vi "System und Gaseinstellung V2 - Kopie.vi"() -> ()   [LabVIEW 2020, in "System Einstellungen V2.lvlib"]
uses:
  System Einstellungen V2.lvlib
  Visualisierungs Elemente/String - Eingabefeld.ctl
  Gasflasche.ctl
  Gasflaschenkomponente.ctl
  Traegergas.ctl
  Aktion FGV Gasbottledefinition.ctl
  Allgemein/allgemeine Sub-VIs.lvlib
panel:
  in  "Update Gas Selects":bool caption="Schaltfläche"
  in  "Registerkartenelement":T1(tab)
  in  "Gasflaschen Liste Pfad":path caption="Gasbottle List File Path"
  in  "Gasflaschen Maske leeren":bool caption="Schaltfläche"
  in  "Gasflasche löschen":bool caption="Schaltfläche"
  in  "Gasflsche einfügen":bool caption="Schaltfläche"
  in  "Gasflasche ändern":bool caption="Schaltfläche"
  in  "Trägergas":T2="N2" caption="Carrier Gas"
  in  "Komponente 5":T3={"Gasauswahl"="", "Konzentration SOLL"=0.0, "Konzentration IST"=0.0, "Einheit"="ppm", "Genauigkeit"=0.0} caption="Component 5" {"Konzentration SOLL" format="%#.4f"; "Konzentration IST" format="%#.4f"; "Genauigkeit" format="%#.1f"}
  in  "Komponente 4":T3={"Gasauswahl"="", "Konzentration SOLL"=0.0, "Konzentration IST"=0.0, "Einheit"="ppm", "Genauigkeit"=0.0} caption="Component 4" {"Konzentration SOLL" format="%#.4f"; "Konzentration IST" format="%#.4f"; "Genauigkeit" format="%#.1f"}
  in  "Komponente 3":T3={"Gasauswahl"="", "Konzentration SOLL"=0.0, "Konzentration IST"=0.0, "Einheit"="ppm", "Genauigkeit"=0.0} caption="Component 3" {"Konzentration SOLL" format="%#.4f"; "Konzentration IST" format="%#.4f"; "Genauigkeit" format="%#.1f"}
  in  "Komponente 2":T3={"Gasauswahl"="", "Konzentration SOLL"=0.0, "Konzentration IST"=0.0, "Einheit"="ppm", "Genauigkeit"=0.0} caption="Component 2" {"Konzentration SOLL" format="%#.4f"; "Konzentration IST" format="%#.4f"; "Genauigkeit" format="%#.1f"}
  in  "Komponente 1":T3={"Gasauswahl"="", "Konzentration SOLL"=0.0, "Konzentration IST"=0.0, "Einheit"="ppm", "Genauigkeit"=0.0} caption="Component 1" {"Konzentration SOLL" format="%#.4f"; "Konzentration IST" format="%#.4f"; "Genauigkeit" format="%#.1f"}
  in  "Gasflasche":T4={"Gasname für die Auswahl"="CH4", "Gasflaschennummer  (Zylinder)"="D15442589", "Chargennummer"="D15442589", "Volumen"="D15442589", "Herstelldatum"=timestamp(0 s since 1904-01-01), "Ablaufdatum"=timestamp(0 s since 1904-01-01)} {"Ablaufdatum" format="%<%d.%m.%Y>T"; "Herstelldatum" format="%<%d.%m.%Y>T"}
  in  "GF import":bool caption="Schaltfläche 2"
  in  "GF export":bool caption="Schaltfläche"
  in  "Gasflaschen Liste":i32(listbox) caption="List of Gasbottles"
  in  "Gas Eingabe":T5
  in  "Gas einfügen":bool caption="Schaltfläche"
  in  "Markiertes Gas löschen":bool caption="Schaltfläche"
  in  "Gasauswahl":i32(listbox) caption="Gasauswahl erstellte Gasflaschen"
  # "System Settings"
  # "Ziel: bei jeder PDF und Einstellung die Seriennummer automatisch laden oder auszuwählen zu können"
  # "Analysator Seriennummer Eintrag"
  # "Alte Systemeinstellungen (PopUp) übernehmen"
  # "Unsere derzeitige Calgas Einstellung fürs Kalibrieren\n\nEventuell Analyser Spalte wie LowNox"
  # "Gas"
  # "Nominal"
  # "Real"
  # "Unit"
  # "Accuracy %"
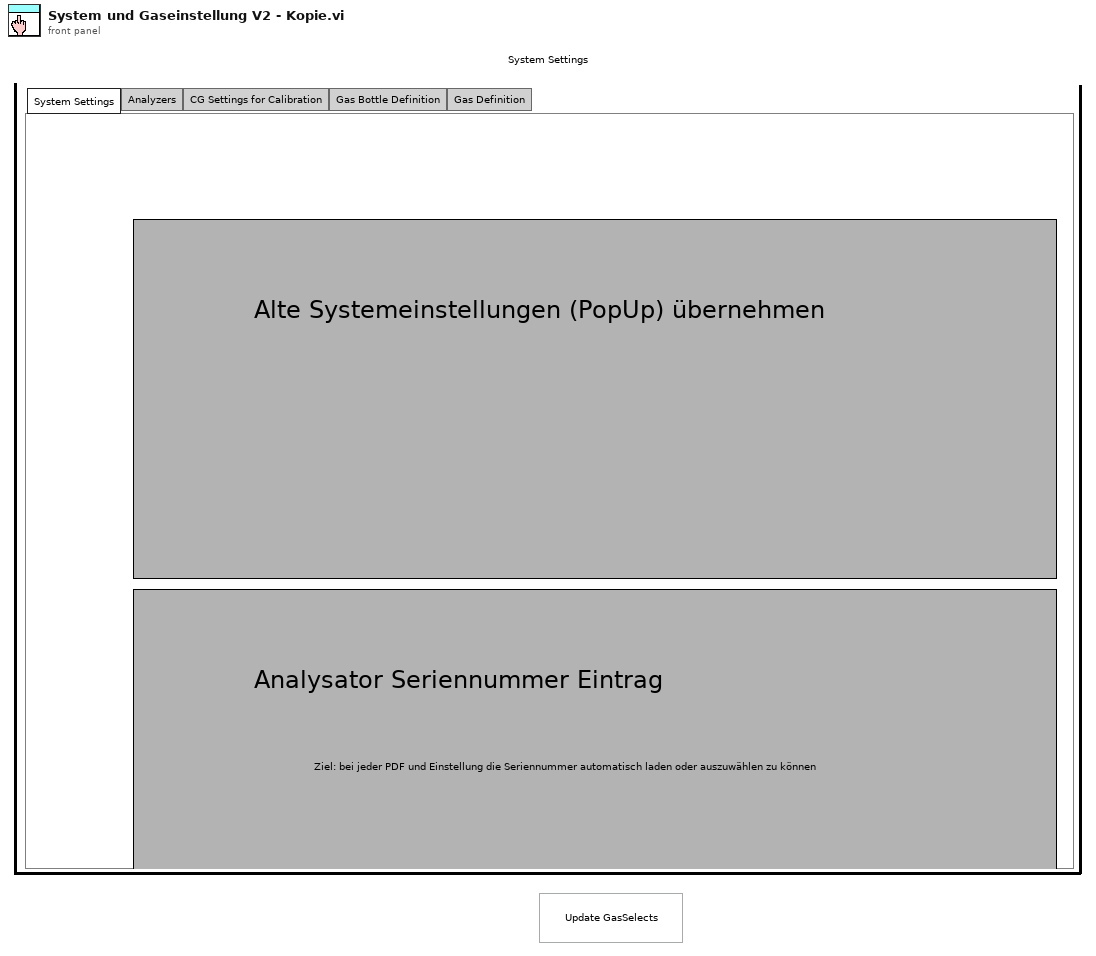
[diagram p1: front panel]
types:
  T1 = enum32{"Systemeinstellungen", "Analysatoren", "CG-Einstellung für Kalibrierung", "Gasflaschenkonfiguration", "Gasdefinition"}
  T2 = typedef "System Einstellungen V2.lvlib/Traegergas.ctl" = string
  T3 = typedef "System Einstellungen V2.lvlib/Gasflaschenkomponente.ctl" = cluster{"Gasauswahl":string, "Konzentration SOLL":dbl, "Konzentration IST":dbl, "Einheit":string, "Genauigkeit":dbl}
  T4 = typedef "System Einstellungen V2.lvlib/Gasflasche.ctl" = cluster{"Gasname für die Auswahl":string, "Gasflaschennummer  (Zylinder)":string, "Chargennummer":string, "Volumen":string, "Herstelldatum":timestamp, "Ablaufdatum":timestamp}
  T5 = typedef "String - Eingabefeld.ctl" = string
  T6 = typedef "Aktion FGV Gasbottledefinition.ctl" = enum16{"lesen", "schreiben", "löschen", "laden", "speichern", "exportieren", "importieren"}
  T7 = enum16{"lesen", "schreiben", "löschen", "laden", "speichern"}
  T8 = typedef "System Einstellungen V2.lvlib/Gasflasche gesamt.ctl" = cluster{"Gasflasche":T4, "Trägergas":T2, "Komponenten":T3[]}
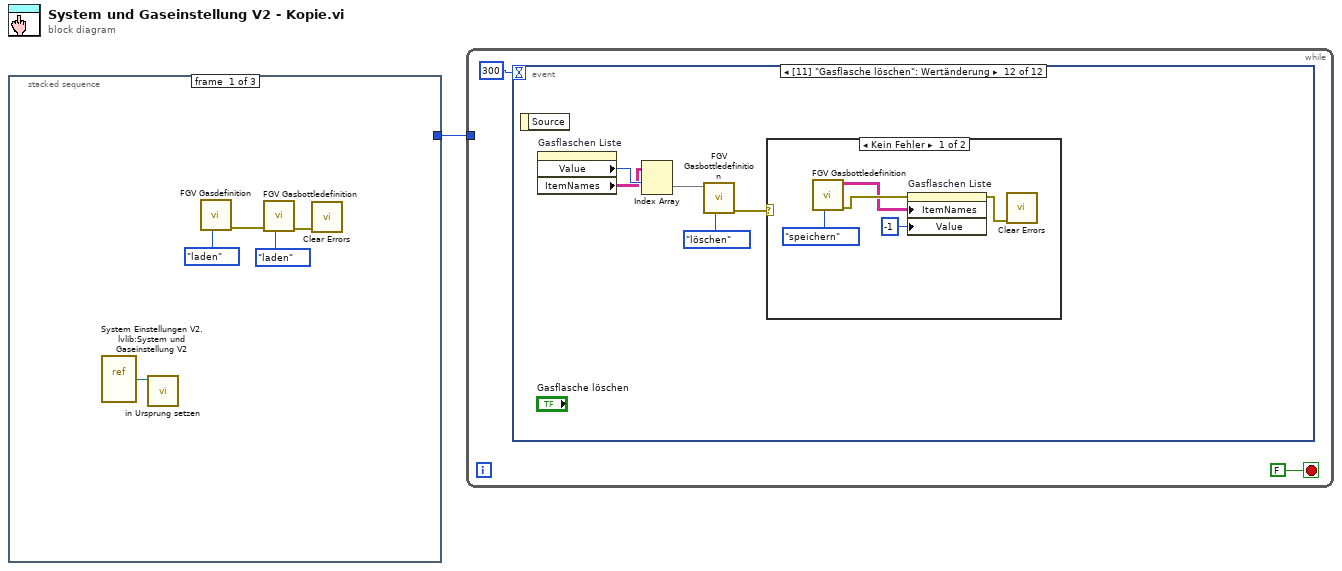
[diagram p0: block diagram]
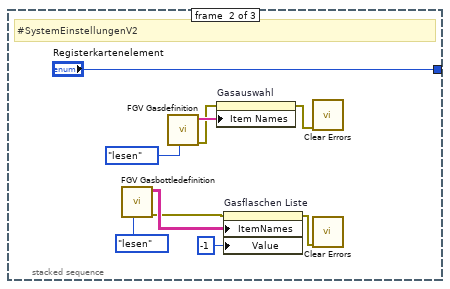
[diagram p2: hidden frame]
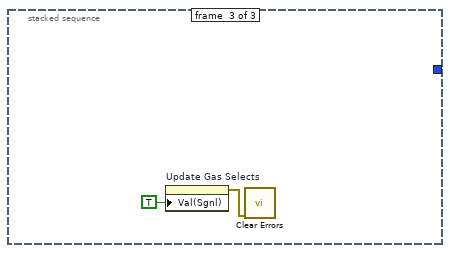
[diagram p3: hidden frame]
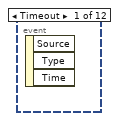
[diagram p4: hidden frame]
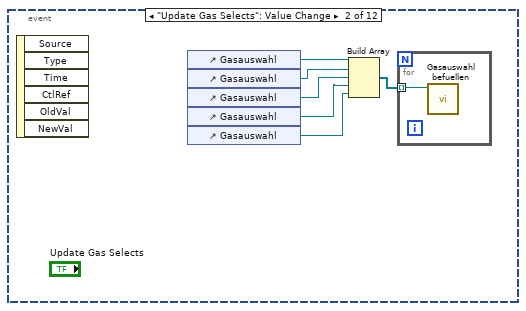
[diagram p5: hidden frame]
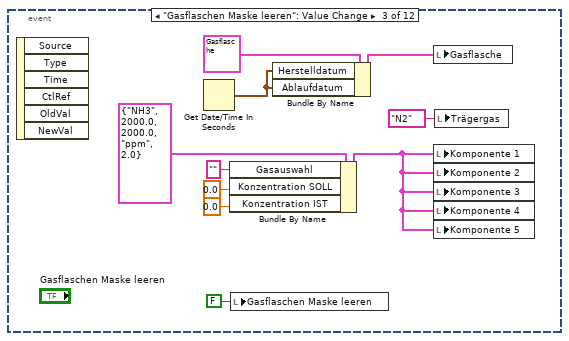
[diagram p6: hidden frame]
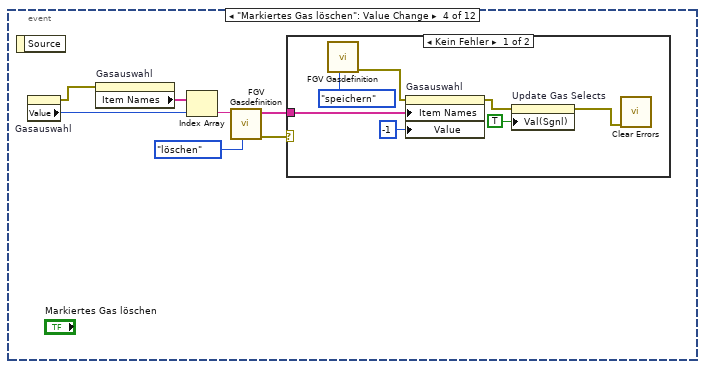
[diagram p7: hidden frame]
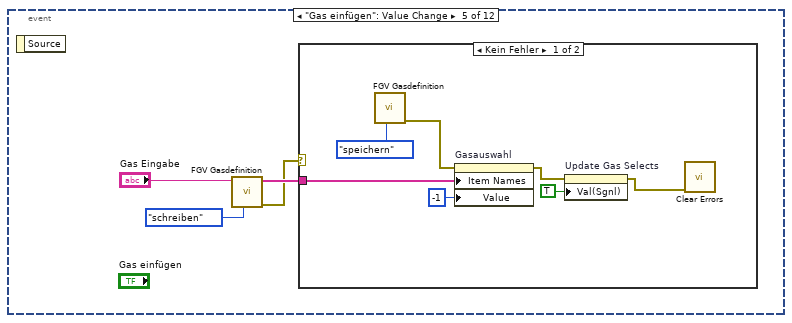
[diagram p9: hidden frame]
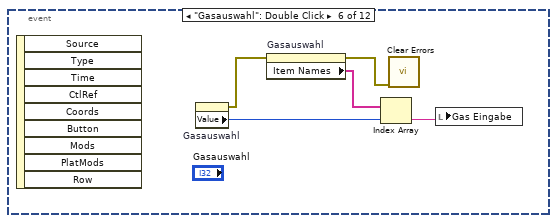
[diagram p11: hidden frame]
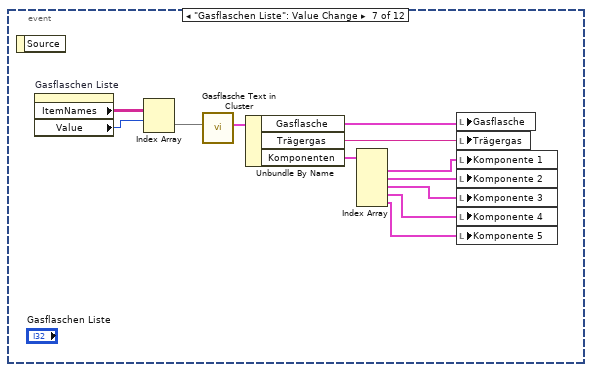
[diagram p12: hidden frame]
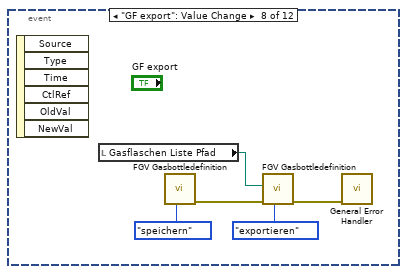
[diagram p13: hidden frame]
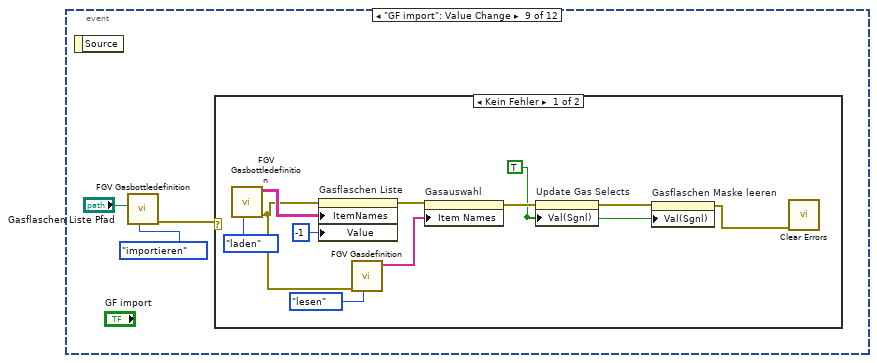
[diagram p14: hidden frame]
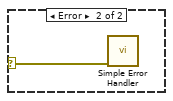
[diagram p15: hidden frame]
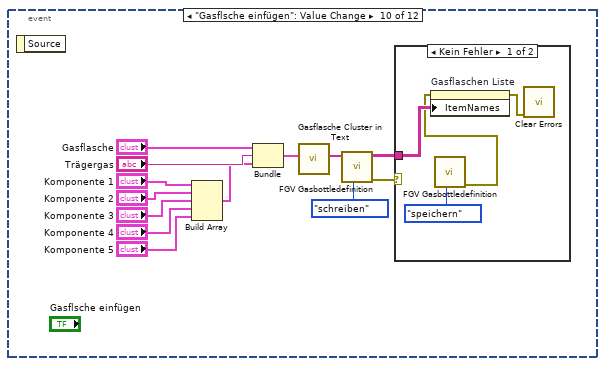
[diagram p16: hidden frame]
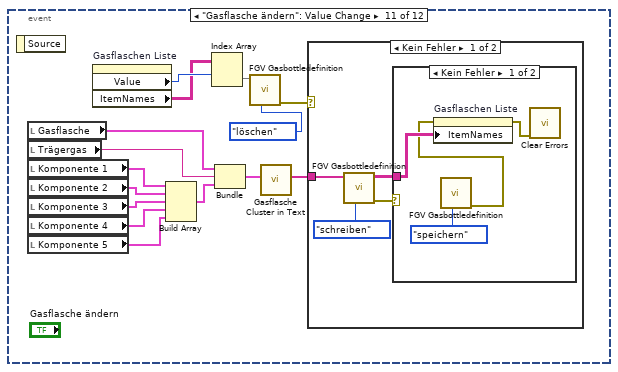
[diagram p18: hidden frame]
diagram:
  n1 = stacked-sequence {
    tunnel: [_ "Registerkartenelement" _] -> w1
    frame #0 {
      n2 = vi-ref "System Einstellungen V2.lvlib:System und Gaseinstellung V2.vi"() -> (w2:refnum<vi>)
      n3 = call "in Ursprung setzen.vi"("VI Referenz"=w2) -> ()  [unwired: 11 in]
      n4 = call "FGV Gasdefinition.vi"("Aktion"=T7."laden") -> ("error out"=w4:errorcluster)  [unwired: 9 in, 1 out]
      n5 = call "FGV Gasbottledefinition.vi"("Aktion"=Aktion_FGV_Gasbottledefinition."laden", "error in (no error)"=w4) -> ("error out"=w3:errorcluster)  [unwired: 7 in, 2 out]
      n6 = call <vilib>:"Clear Errors.vi"("error in (no error)"=w3) -> ()  [unwired: 5 in, 2 out]
    }
    frame #1 {
      # "#SystemEinstellungenV2"
      n7 = call "FGV Gasbottledefinition.vi"("Aktion"=Aktion_FGV_Gasbottledefinition."lesen") -> ("error out"=w10:errorcluster, "Gasflaschen Test Liste gesamt"=w11:T2[][])  [unwired: 8 in, 1 out]
      n8 = call "FGV Gasdefinition.vi"("Aktion"=T7."lesen") -> ("error out"=w8:errorcluster, "Gase"=w14:string[])  [unwired: 9 in]
      n9 = property on="Gasauswahl" class="Listenfeld (strikt)"(error in=w8, "Item Names"=w14) -> (error out=w13:errorcluster)  [unwired: 1 in, 1 out]
      n10 = property on="Gasflaschen Liste" class="MehrSpaltFeld (strikt)"(error in=w10, "ItemNames"=w11, "Value"=-1 ("Gasflaschen Liste")) -> (error out=w9:errorcluster)  [unwired: 1 in, 1 out]
      n11 = call <vilib>:"Clear Errors.vi"("error in (no error)"=w13) -> ()  [unwired: 5 in, 2 out]
      n12 = call <vilib>:"Clear Errors.vi"("error in (no error)"=w9) -> ()  [unwired: 5 in, 2 out]
    }
    frame #2 {
      n13 = property on="Update Gas Selects" class="Bool. (strikt)"("Val(Sgnl)"=TRUE ("Wert (signalisierend)")) -> (error out=w18:errorcluster)  [unwired: 2 in, 1 out]
      n14 = call <vilib>:"Clear Errors.vi"("error in (no error)"=w18) -> ()  [unwired: 5 in, 2 out]
    }
  }
  n15 = while {
    tunnel: w1 -> [_]
    stop <- FALSE stop-if-true
    n16 = event shown="[11] \"Gasflasche löschen\": Wertänderung" {
      selector: _ -> [_ _ _ _ _ _ _ _ _ _ _ _]
      dyn-events: _ -> [_ _ _ _ _ _ _ _ _ _ _ _]
      timeout: 300 -> [_ _ _ _ _ _ _ _ _ _ _ _]
      event Timeout {
        n17 = event-data() -> ()  [unwired: 1 in, 3 out]
      }
      event "Update Gas Selects": Value Change {
        n18 = event-data() -> ()  [unwired: 1 in, 6 out]
        n19 = control-ref of="Gasauswahl"() -> (w21:refnum<vi>)
        n20 = control-ref of="Gasauswahl"() -> (w22:refnum<vi>)
        n21 = control-ref of="Gasauswahl"() -> (w23:refnum<vi>)
        n22 = control-ref of="Gasauswahl"() -> (w24:refnum<vi>)
        n23 = control-ref of="Gasauswahl"() -> (w25:refnum<vi>)
        n24 = Build Array(w21, w22, w23, w24, w25) -> (w26:refnum<vi>[])
        n25 = for {
          tunnel: w26 -> [w27] mode=indexing
          n26 = call "Gasauswahl befuellen.vi"("Kombinationsfeld (Eingang)"=w27) -> ()  [unwired: 11 in]
        }
      }
      event "Gasflaschen Maske leeren": Value Change {
        n27 = event-data() -> ()  [unwired: 1 in, 6 out]
        n28 = Get Date/Time In Seconds() -> (seconds since 1Jan1904=w30:timestamp)
        n29 = Bundle By Name(cluster=T3 {"Gasauswahl"="NH3", "Konzentration SOLL"=2000.0, "Konzentration IST"=2000.0, "Einheit"="ppm", "Genauigkeit"=2.0} ("Komponente 1"), "Gasauswahl"="", "Konzentration SOLL"=0.0, "Konzentration IST"=0.0) -> (w32:T3)
        n30 = local write "Gasflaschen Maske leeren"(FALSE ("Gasflaschen Maske leeren")) -> ()
        n31 = Bundle By Name(cluster=T4 {"Gasname für die Auswahl"="", "Gasflaschennummer  (Zylinder)"="", "Chargennummer"="", "Volumen"="", "Herstelldatum"=timestamp(3692908800 s since 1904-01-01), "Ablaufdatum"=timestamp(3724444800 s since 1904-01-01)} ("Gasflasche"), "Herstelldatum"=w30, "Ablaufdatum"=w30) -> (w31:T4)
        n32 = local write "Gasflasche"(w31) -> ()
        n33 = local write "Komponente 1"(w32) -> ()
        n34 = local write "Komponente 2"(w32) -> ()
        n35 = local write "Komponente 3"(w32) -> ()
        n36 = local write "Komponente 4"(w32) -> ()
        n37 = local write "Komponente 5"(w32) -> ()
        n38 = local write "Trägergas"(T2 "N2" ("Trägergas")) -> ()
      }
      event "Markiertes Gas löschen": Value Change {
        n39 = event-data() -> ()  [unwired: 1 in, 1 out]
        n40 = property on="Gasauswahl" class="Listenfeld (strikt)"() -> (error out=w40:errorcluster, "Value"=w42:i32)  [unwired: 2 in, 1 out]
        n41 = property on="Gasauswahl" class="Listenfeld (strikt)"(error in=w40) -> ("Item Names"=w43:string[])  [unwired: 1 in, 2 out]
        n42 = Index Array(array=w43, index=w42) -> (element=w41:string)
        n43 = call "FGV Gasdefinition.vi"("Aktion"=T7."löschen", "Gas"=w41) -> ("error out"=w38:errorcluster, "Gase"=w39:string[])  [unwired: 8 in]
        n44 = case shown="Kein Fehler" w38 {
          tunnel: w39 -> [w51 _]
          frame No Error {
            n45 = call "FGV Gasdefinition.vi"("Aktion"=T7."speichern") -> ("error out"=w48:errorcluster)  [unwired: 9 in, 1 out]
            n46 = property on="Gasauswahl" class="Listenfeld (strikt)"(error in=w48, "Item Names"=w51, "Value"=-1 ("Gasauswahl")) -> (error out=w47:errorcluster)  [unwired: 1 in, 1 out]
            n47 = property on="Update Gas Selects" class="Bool. (strikt)"(error in=w47, "Val(Sgnl)"=TRUE ("Wert (signalisierend)")) -> (error out=w46:errorcluster)  [unwired: 1 in, 1 out]
            n48 = call <vilib>:"Clear Errors.vi"("error in (no error)"=w46) -> ()  [unwired: 5 in, 2 out]
          }
          frame Error {
          }
        }
      }
      event "Gas einfügen": Value Change {
        n49 = event-data() -> ()  [unwired: 1 in, 1 out]
        n50 = call "FGV Gasdefinition.vi"("Aktion"=T7."schreiben", "Gas"="Gas Eingabe") -> ("error out"=w52:errorcluster, "Gase"=w53:string[])  [unwired: 8 in]
        n51 = case shown="Kein Fehler" w52 {
          tunnel: w53 -> [w62 _]
          frame No Error {
            n52 = call "FGV Gasdefinition.vi"("Aktion"=T7."speichern") -> ("error out"=w59:errorcluster)  [unwired: 9 in, 1 out]
            n53 = property on="Gasauswahl" class="Listenfeld (strikt)"(error in=w59, "Item Names"=w62, "Value"=-1 ("Gasauswahl")) -> (error out=w58:errorcluster)  [unwired: 1 in, 1 out]
            n54 = property on="Update Gas Selects" class="Bool. (strikt)"(error in=w58, "Val(Sgnl)"=TRUE ("Wert (signalisierend)")) -> (error out=w57:errorcluster)  [unwired: 1 in, 1 out]
            n55 = call <vilib>:"Clear Errors.vi"("error in (no error)"=w57) -> ()  [unwired: 5 in, 2 out]
          }
          frame Error {
          }
        }
      }
      event "Gasauswahl": Double Click {
        n56 = event-data() -> ()  [unwired: 1 in, 9 out]
        n57 = property on="Gasauswahl" class="Listenfeld (strikt)"() -> (error out=w64:errorcluster, "Value"=w66:i32)  [unwired: 2 in, 1 out]
        n58 = property on="Gasauswahl" class="Listenfeld (strikt)"(error in=w64) -> (error out=w63:errorcluster, "Item Names"=w67:string[])  [unwired: 1 in, 1 out]
        n59 = Index Array(array=w67, index=w66) -> (element=w65:string)
        n60 = call <vilib>:"Clear Errors.vi"("error in (no error)"=w63) -> ()  [unwired: 5 in, 2 out]
        n61 = local write "Gas Eingabe"(w65) -> ()
      }
      event "Gasflaschen Liste": Value Change {
        n62 = event-data() -> ()  [unwired: 1 in, 1 out]
        n63 = property on="Gasflaschen Liste" class="MehrSpaltFeld (strikt)"() -> ("ItemNames"=w79:string[][], "Value"=w78:i32)  [unwired: 2 in, 2 out]
        n64 = Index Array(array=w79, index (row)=w78) -> (element=w77:string[])  [unwired: 1 in]
        n65 = call "Gasflasche Text in Cluster.vi"("Gasflasche Text Array"=w77) -> ("Gasflasche"=w76:T8)  [unwired: 10 in]
        n66 = Unbundle By Name(w76) -> ("Gasflasche"=w75:T4, "Trägergas"=w74:T2, "Komponenten"=w73:T3[])
        n67 = Index Array(array=w73) -> (element #1=w72:T3, element #2=w71:T3, element #3=w70:T3, element #4=w69:T3, element #5=w68:T3)  [unwired: 5 in]
        n68 = local write "Gasflasche"(w75) -> ()
        n69 = local write "Trägergas"(w74) -> ()
        n70 = local write "Komponente 1"(w72) -> ()
        n71 = local write "Komponente 2"(w71) -> ()
        n72 = local write "Komponente 3"(w70) -> ()
        n73 = local write "Komponente 4"(w69) -> ()
        n74 = local write "Komponente 5"(w68) -> ()
      }
      event "GF export": Value Change {
        n75 = event-data() -> ()  [unwired: 1 in, 6 out]
        n76 = local read "Gasflaschen Liste Pfad"() -> (w80:path)
        n77 = call "FGV Gasbottledefinition.vi"("Aktion"=Aktion_FGV_Gasbottledefinition."speichern") -> ("error out"=w82:errorcluster)  [unwired: 8 in, 2 out]
        n78 = call "FGV Gasbottledefinition.vi"("Aktion"=Aktion_FGV_Gasbottledefinition."exportieren", "error in (no error)"=w82, "Dateipfad"=w80) -> ("error out"=w81:errorcluster)  [unwired: 6 in, 2 out]
        n79 = call <vilib>:"General Error Handler.vi"("error in (no error)"=w81) -> ()  [unwired: 10 in, 5 out]
      }
      event "GF import": Value Change {
        n80 = event-data() -> ()  [unwired: 1 in, 1 out]
        n81 = call "FGV Gasbottledefinition.vi"("Aktion"=Aktion_FGV_Gasbottledefinition."importieren", "Dateipfad"="Gasflaschen Liste Pfad") -> ("error out"=w85:errorcluster)  [unwired: 7 in, 2 out]
        n82 = case shown="Kein Fehler" w85 {
          selector: w85 -> [_ w99]
          frame No Error {
            w91 = TRUE ("Wert (signalisierend)")
            n83 = call "FGV Gasbottledefinition.vi"("Aktion"=Aktion_FGV_Gasbottledefinition."laden") -> ("error out"=w88:errorcluster, "Gasflaschen Test Liste gesamt"=w97:T2[][])  [unwired: 8 in, 1 out]
            n84 = property on="Gasflaschen Liste" class="MehrSpaltFeld (strikt)"(error in=w88, "ItemNames"=w97, "Value"=-1 ("Gasflaschen Liste")) -> (error out=w93:errorcluster)  [unwired: 1 in, 1 out]
            n85 = call "FGV Gasdefinition.vi"("Aktion"=T7."lesen", "error in (no error)"=w88) -> ("Gase"=w94:string[])  [unwired: 8 in, 1 out]
            n86 = property on="Gasauswahl" class="Listenfeld (strikt)"(error in=w93, "Item Names"=w94) -> (error out=w92:errorcluster)  [unwired: 1 in, 1 out]
            n87 = property on="Update Gas Selects" class="Bool. (strikt)"(error in=w92, "Val(Sgnl)"=w91) -> (error out=w90:errorcluster)  [unwired: 1 in, 1 out]
            n88 = property on="Gasflaschen Maske leeren" class="Bool. (strikt)"(error in=w90, "Val(Sgnl)"=w91) -> (error out=w89:errorcluster)  [unwired: 1 in, 1 out]
            n89 = call <vilib>:"Clear Errors.vi"("error in (no error)"=w89) -> ()  [unwired: 5 in, 2 out]
          }
          frame Error {
            n90 = call <vilib>:"Simple Error Handler.vi"("error in (no error)"=w99) -> ()  [unwired: 4 in, 5 out]
          }
        }
      }
      event "Gasflsche einfügen": Value Change {
        n91 = event-data() -> ()  [unwired: 1 in, 1 out]
        n92 = Build Array("Komponente 1", "Komponente 2", "Komponente 3", "Komponente 4", "Komponente 5") -> (w105:T3[])
        n93 = Bundle("Gasflasche"="Gasflasche", "Trägergas"="Trägergas", w105) -> (w104:cluster{"Gasflasche":T4, "Trägergas":T2, T3[]})  [unwired: 1 in]
        n94 = call "Gasflasche Cluster in Text.vi"("Gasflasche"=w104) -> ("Gasflasche Text Array"=w102:T2[])  [unwired: 10 in]
        n95 = call "FGV Gasbottledefinition.vi"("Aktion"=Aktion_FGV_Gasbottledefinition."schreiben", "Gasflasche Text Array"=w102) -> ("error out"=w100:errorcluster, "Gasflaschen Test Liste gesamt"=w101:T2[][])  [unwired: 7 in, 1 out]
        n96 = case shown="Kein Fehler" w100 {
          tunnel: w101 -> [w115 _]
          frame No Error {
            n97 = call "FGV Gasbottledefinition.vi"("Aktion"=Aktion_FGV_Gasbottledefinition."speichern") -> ("error out"=w113:errorcluster)  [unwired: 8 in, 2 out]
            n98 = property on="Gasflaschen Liste" class="MehrSpaltFeld (strikt)"(error in=w113, "ItemNames"=w115) -> (error out=w114:errorcluster)  [unwired: 1 in, 1 out]
            n99 = call <vilib>:"Clear Errors.vi"("error in (no error)"=w114) -> ()  [unwired: 5 in, 2 out]
          }
          frame Error {
          }
        }
      }
      event "Gasflasche ändern": Value Change {
        n100 = event-data() -> ()  [unwired: 1 in, 1 out]
        n101 = local read "Gasflasche"() -> (w129:T4)
        n102 = local read "Trägergas"() -> (w128:T2)
        n103 = local read "Komponente 1"() -> (w127:T3)
        n104 = local read "Komponente 2"() -> (w126:T3)
        n105 = local read "Komponente 3"() -> (w125:T3)
        n106 = local read "Komponente 4"() -> (w124:T3)
        n107 = local read "Komponente 5"() -> (w123:T3)
        n108 = property on="Gasflaschen Liste" class="MehrSpaltFeld (strikt)"() -> ("Value"=w120:i32, "ItemNames"=w119:string[][])  [unwired: 2 in, 2 out]
        n109 = Build Array(w127, w126, w125, w124, w123) -> (w122:T3[])
        n110 = Index Array(array=w119, index (row)=w120) -> (element=w121:string[])  [unwired: 1 in]
        n111 = Bundle("Gasflasche"=w129, "Trägergas"=w128, w122) -> (w131:cluster{"Gasflasche":T4, "Trägergas":T2, T3[]})  [unwired: 1 in]
        n112 = call "FGV Gasbottledefinition.vi"("Aktion"=T7."löschen", "Gasflasche Text Array"=w121) -> ("error out"=w117:errorcluster)  [unwired: 7 in, 2 out]
        n113 = call "Gasflasche Cluster in Text.vi"("Gasflasche"=w131) -> ("Gasflasche Text Array"=w130:T2[])  [unwired: 10 in]
        n114 = case shown="Kein Fehler" w117 {
          tunnel: w130 -> [w135 _]
          frame No Error {
            n115 = call "FGV Gasbottledefinition.vi"("Aktion"=Aktion_FGV_Gasbottledefinition."schreiben", "Gasflasche Text Array"=w135) -> ("error out"=w133:errorcluster, "Gasflaschen Test Liste gesamt"=w134:T2[][])  [unwired: 7 in, 1 out]
            n116 = case shown="Kein Fehler" w133 {
              tunnel: w134 -> [w138 _]
              frame No Error {
                n117 = call "FGV Gasbottledefinition.vi"("Aktion"=Aktion_FGV_Gasbottledefinition."speichern") -> ("error out"=w137:errorcluster)  [unwired: 8 in, 2 out]
                n118 = property on="Gasflaschen Liste" class="MehrSpaltFeld (strikt)"(error in=w137, "ItemNames"=w138) -> (error out=w136:errorcluster)  [unwired: 1 in, 1 out]
                n119 = call <vilib>:"Clear Errors.vi"("error in (no error)"=w136) -> ()  [unwired: 5 in, 2 out]
              }
              frame Error {
              }
            }
          }
          frame Error {
          }
        }
      }
      event "Gasflasche löschen": Value Change {
        n120 = event-data() -> ()  [unwired: 1 in, 1 out]
        n121 = property on="Gasflaschen Liste" class="MehrSpaltFeld (strikt)"() -> ("Value"=w144:i32, "ItemNames"=w143:string[][])  [unwired: 2 in, 2 out]
        n122 = Index Array(array=w143, index (row)=w144) -> (element=w141:string[])  [unwired: 1 in]
        n123 = call "FGV Gasbottledefinition.vi"("Aktion"=Aktion_FGV_Gasbottledefinition."löschen", "Gasflasche Text Array"=w141) -> ("error out"=w140:errorcluster)  [unwired: 7 in, 2 out]
        n124 = case shown="Kein Fehler" w140 {
          frame No Error {
            n125 = call "FGV Gasbottledefinition.vi"("Aktion"=Aktion_FGV_Gasbottledefinition."speichern") -> ("error out"=w148:errorcluster, "Gasflaschen Test Liste gesamt"=w147:T2[][])  [unwired: 8 in, 1 out]
            n126 = property on="Gasflaschen Liste" class="MehrSpaltFeld (strikt)"(error in=w148, "ItemNames"=w147, "Value"=-1 ("Gasflaschen Liste")) -> (error out=w146:errorcluster)  [unwired: 1 in, 1 out]
            n127 = call <vilib>:"Clear Errors.vi"("error in (no error)"=w146) -> ()  [unwired: 5 in, 2 out]
          }
          frame Error {
          }
        }
      }
    }
  }
